vi "Get Cursor Positions.vi"(8 "Error In":errorcluster, 11 "XYGraph in":refnum<vi>) -> (0 "Error Out":errorcluster, 1 "Cursor 1-3 Positions":dbl[](array[numeric]), 2 "Cursor 1 & 2 Positions":dbl[](array[numeric]), 3 "Cursor 1 Position":dbl)   [LabVIEW 2019]
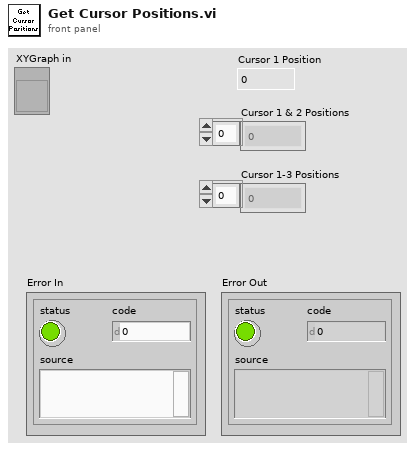
[diagram p1: front panel]
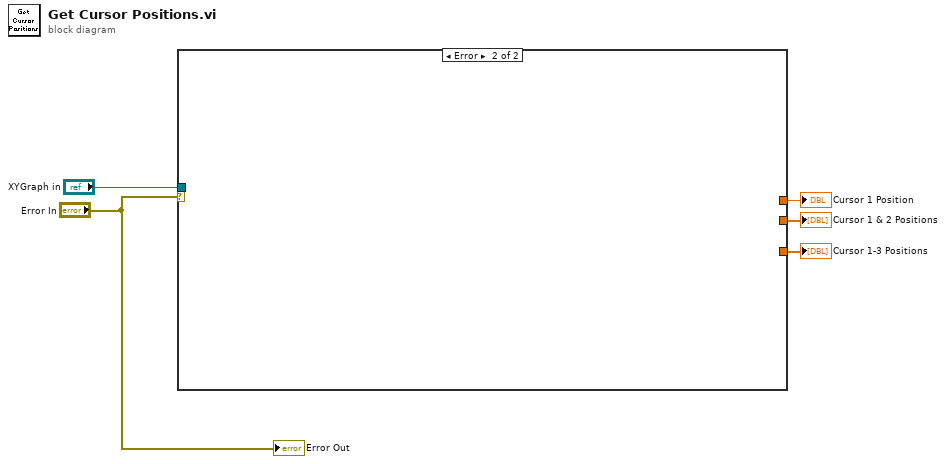
[diagram p0: block diagram]
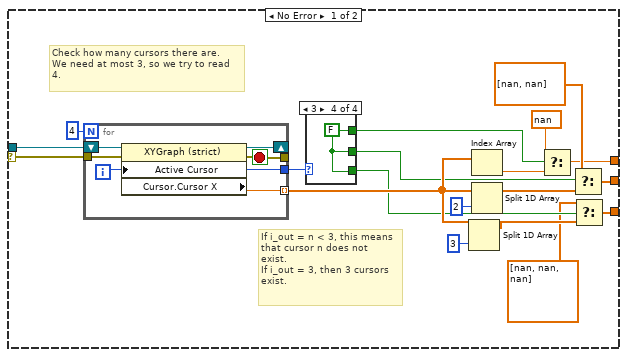
[diagram p2: hidden frame]
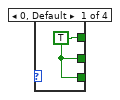
[diagram p3: hidden frame]
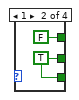
[diagram p4: hidden frame]
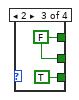
[diagram p5: hidden frame]
diagram:
  n1 = case shown="Error" "Error In" {
    selector: "Error In" -> [w6 _]
    tunnel: [w10 _] -> w5
    tunnel: [w9 _] -> w4
    tunnel: [w8 _] -> w3
    tunnel: "XYGraph in" -> [w7 _]
    frame No Error {
      # "If i_out = n < 3, this means\nthat cursor n does not\nexist.\nIf i_out = 3, then 3 cursors\nexist."
      # "Check how many cursors there are.\nWe need at most 3, so we try to read\n4."
      n2 = for {
        N: u32 4 ("Active Cursor") -> [_]
        tunnel: [w33] -> w22 mode=indexing
        shift-right: [w34] -> _
        shift-left: w7 -> [w36]
        tunnel: w6 -> [w35]
        tunnel: [w32] -> w17
        tunnel: [w31] -> _
        i -> [w32]
        stop <- w31 stop-if-true
        n3 = property class="XYGraph (strict)"(reference=w36, error in=w35, "Active Cursor"=w32) -> (reference out=w34:refnum<vi>, error out=w31:errorcluster, "Cursor.Cursor X"=w33:dbl)
      }
      n4 = case shown="3" w17 {
        tunnel: [w25 FALSE ("s") w28 w30] -> w18
        tunnel: [w25 w26 w28 w30] -> w19
        tunnel: [w25 w26 TRUE ("s") w30] -> w20
        frame 0, Default {
          w25 = TRUE ("s")
        }
        frame 1 {
          w26 = TRUE ("s")
        }
        frame 2 {
          w28 = FALSE ("s")
        }
        frame 3 {
          w30 = FALSE ("s")
        }
      }
      n5 = Split 1D Array(array=w22, index=3) -> (first subarray=w23:dbl[])  [unwired: 1 out]
      n6 = Index Array(array=w22) -> (element=w16:dbl)  [unwired: 1 in]
      n7 = Split 1D Array(array=w22, index=2) -> (first subarray=w21:dbl[])  [unwired: 1 out]
      n8 = Select(t=nan, s=w18, f=w16) -> (s? t:f=w8:dbl)
      n9 = Select(t=dbl[] [nan, nan], s=w19, f=w21) -> (s? t:f=w9:dbl[])
      n10 = Select(t=dbl[] [nan, nan, nan], s=w20, f=w23) -> (s? t:f=w10:dbl[])
    }
    frame Error {
    }
  }
  "Cursor 1-3 Positions" <- w5
  "Cursor 1 & 2 Positions" <- w4
  "Cursor 1 Position" <- w3
  "Error Out" <- "Error In"
